vi "Update Package Version.vi"(8 "error in (no error)":errorcluster, 11 "Build Package Step in":refnum<class "Build Package Step.lvclass">) -> (0 "error out":errorcluster, 3 "Build Package Step out":refnum<class "Build Package Step.lvclass">)   [LabVIEW 2019, in "VIPM.lvlib" / "Build Package Step.lvclass"]
uses:
  Build Package Step.lvclass
  <vilib>/JKI/VIPM API/VIPM API_vipm_api.lvlib
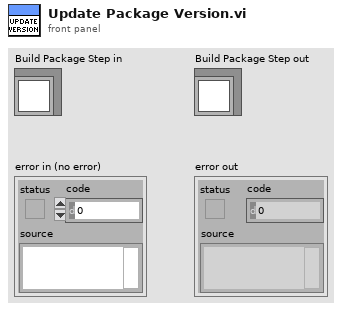
[diagram p1: front panel]
types:
  T1 = typedef "Solution.lvlibp/Build Step.lvclass/Build Settings.ctl" = cluster{"Force?":bool, "Version":T2}
  T2 = typedef "Solution.lvlibp/Version.ctl" = cluster{"Major":i32, "Minor":i32, "Build":i32, "Patch":i32}
  T3 = typedef "VIPM API_vipm_api.lvlib/VI Package Build Spec Data Cluster_vipm_api.ctl" = cluster{"Package Version":T4, "Product Name":string, "Company Name":string, "Author Name (Person or Company)":string, "Product Homepage (URL)":string, "Legal Copyright":string, "License Agreement Name":string, "Product Description Summary":string, "Product Description":string, "Release Notes - Change Log":string}
  T4 = typedef "VIPM API_vipm_api.lvlib/Version Info Cluster_vipm_api.ctl" = cluster{"major":u32, "minor":u32, "patch":u32, "build":u32}
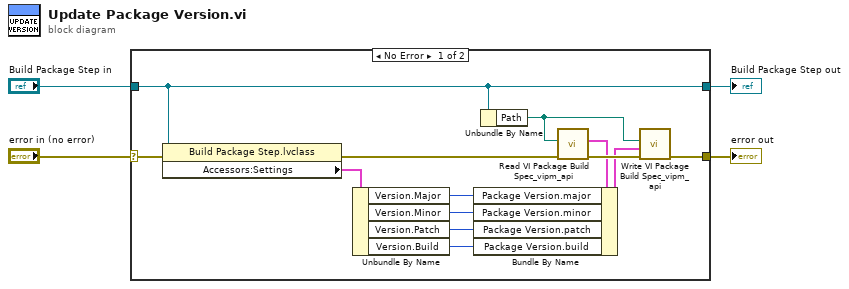
[diagram p0: block diagram]
diagram:
  n1 = case shown="No Error" "error in (no error)" {
    selector: "error in (no error)" -> [w17 w19]
    tunnel: [w15 w19] -> w3
    tunnel: [w13 w18] -> w1
    tunnel: "Build Package Step in" -> [w13 w18]
    frame No Error {
      n2 = property class="Build Package Step.lvclass"(reference=w13, error in=w17) -> (error out=w14:errorcluster, "Accessors:Settings"=w9:T1)  [unwired: 1 out]
      n3 = Unbundle By Name(w9) -> ("Version.Major"=w8:i32, "Version.Minor"=w7:i32, "Version.Patch"=w6:i32, "Version.Build"=w5:i32)
      n4 = Unbundle By Name(w13) -> ("Path"=w10:path)
      n5 = call <vilib>:"Read VI Package Build Spec_vipm_api.vi"("error in (no error)"=w14, "Path to VIPB File"=w10) -> ("error out"=w16:errorcluster, "VI Package Build Spec Data"=w12:T3)  [unwired: 8 in]
      n6 = Bundle By Name(cluster=w12, "Package Version.major"=w8, "Package Version.minor"=w7, "Package Version.patch"=w6, "Package Version.build"=w5) -> (w11:T3)
      n7 = call <vilib>:"Write VI Package Build Spec_vipm_api.vi"("error in (no error)"=w16, "VI Package Build Spec Data"=w11, "Path to VIPB File"=w10) -> ("error out"=w15:errorcluster)  [unwired: 8 in]
    }
    frame Error {
    }
  }
  "error out" <- w3
  "Build Package Step out" <- w1
